vi "UI(Edit_Init).vi"(10 "Map":T1 {"TaskConfig"."SampleRateConfiguration"."SampleMode" items=["Finite Samples"=10178, "Continuous Samples"=10123, "Hardware Timed Single Point"=12522]}, 11 "Listbox":refnum<vi>) -> ()   [LabVIEW 2025, in "DAQ_Module.lvlib" / "DAQ_Module.lvclass"]
uses:
  DAQ_Module.lvclass
  DAQ_Config.ctl
  DAQ_Task_Config.ctl
  DAQ_HW_Type.ctl
  DAQ_Task_Type.ctl
  DAQ_SampleRateConfig.ctl
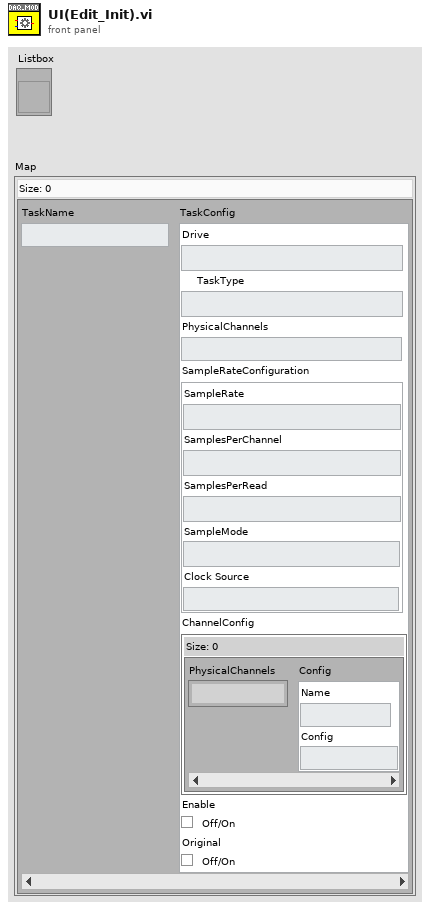
[diagram p1: front panel]
types:
  T1 = typedef "DAQ_Module.lvlib/DAQ_Module.lvclass/DAQ_Config.ctl" = map{string, T2}
  T2 = typedef "DAQ_Module.lvlib/DAQ_Module.lvclass/DAQ_Task_Config.ctl" = cluster{"Drive":T3, "TaskType":T4, "PhysicalChannels":string, "SampleRateConfiguration":T5, "ChannelConfig":map{string, cluster{"Name":string, "Config":string}}, "Enable":bool, "Original":bool}
  T3 = typedef "DAQ_Module.lvlib/DAQ_Module.lvclass/DAQ_HW_Type.ctl" = enum16{"NI_DAQmx", "Simulated_DAQ"}
  T4 = typedef "DAQ_Module.lvlib/DAQ_Module.lvclass/DAQ_Task_Type.ctl" = enum16{"AI", "Linear", "Angular", "AO"}
  T5 = typedef "DAQ_Module.lvlib/DAQ_Module.lvclass/DAQ_SampleRateConfig.ctl" = cluster{"SampleRate":dbl, "SamplesPerChannel":u32, "SamplesPerRead":i32, "SampleMode":i32, "Clock Source":string}
  T6 = cluster{"Left Cell String":string, "Child Text":string[], "Child Tag":string, "Item Indent":i32, "Child Only?":bool, "Glyph Index":i32}
  T7 = map{string, cluster{"Name":string, "Config":string}}
  T8 = cluster{"Left Cell String":string, "Child Text":string[], "Child Tag":string, "Item Indent":i32, "Child Only?":bool, "Glyph Index":i32}[]
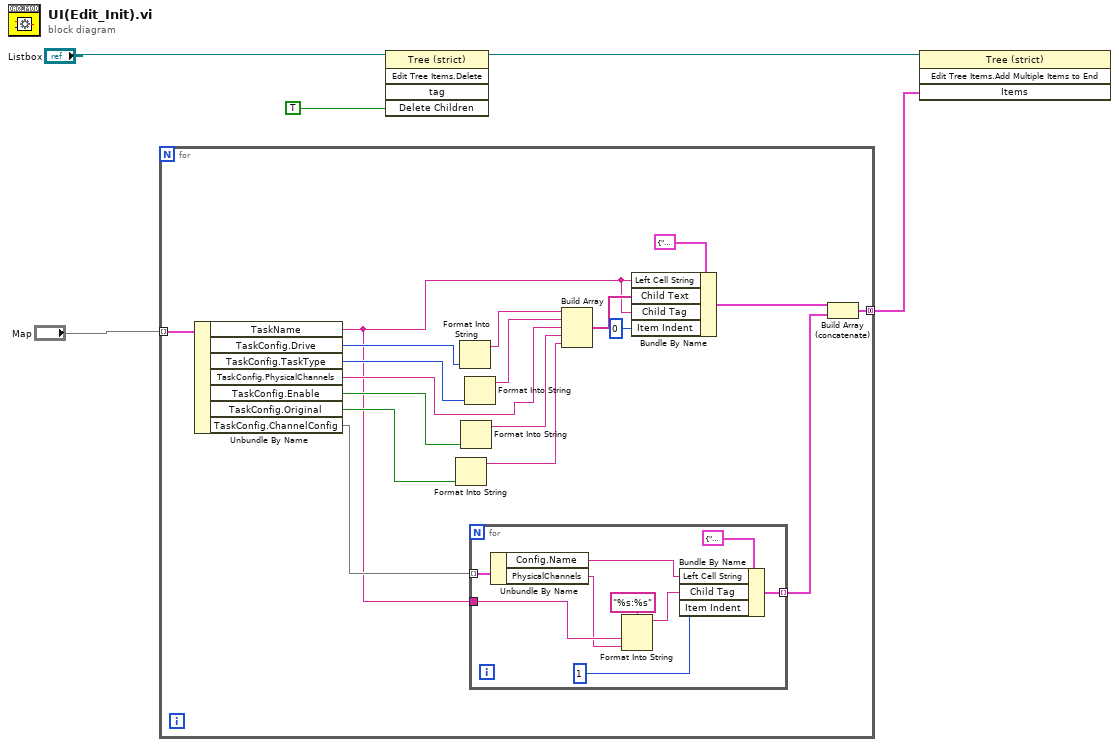
[diagram p0: block diagram]
diagram:
  n1 = for {
    tunnel: "Map" -> [w23] mode=indexing
    tunnel: [w6] -> w2 mode=concatenating
    n2 = Unbundle By Name(w23) -> ("TaskName"=w9:string, "TaskConfig.Drive"=w22:T3, "TaskConfig.TaskType"=w21:T4, "TaskConfig.PhysicalChannels"=w17:string, "TaskConfig.Enable"=w20:bool, "TaskConfig.Original"=w15:bool, "TaskConfig.ChannelConfig"=w11:T7)
    n3 = Format Into String(w15) -> (resulting string=w14:string)  [unwired: 3 in, 1 out]
    n4 = Format Into String(w22) -> (resulting string=w19:string)  [unwired: 3 in, 1 out]
    n5 = Format Into String(w20) -> (resulting string=w16:string)  [unwired: 3 in, 1 out]
    n6 = Format Into String(w21) -> (resulting string=w18:string)  [unwired: 3 in, 1 out]
    n7 = for {
      tunnel: w11 -> [w32] mode=indexing
      tunnel: w9 -> [w28]
      tunnel: [w25] -> w7 mode=indexing
      n8 = Unbundle By Name(w32) -> ("Config.Name"=w24:string, "PhysicalChannels"=w27:string)
      n9 = Format Into String(format string="%s:%s", w28, w27) -> (resulting string=w26:string)  [unwired: 2 in, 1 out]
      n10 = Bundle By Name(cluster=T6 {"Left Cell String"="", "Child Text"=[], "Child Tag"="", "Item Indent"=0, "Child Only?"=FALSE, "Glyph Index"=0} ("Item"), "Left Cell String"=w24, "Child Tag"=w26, "Item Indent"=1) -> (w25:T6)
    }
    n11 = Build Array(w19, w18, w17, w16, w14) -> (w12:string[])
    n12 = Bundle By Name(cluster=T6 {"Left Cell String"="", "Child Text"=[], "Child Tag"="", "Item Indent"=0, "Child Only?"=FALSE, "Glyph Index"=0} ("Item"), "Left Cell String"=w9, "Child Text"=w12, "Child Tag"=w9, "Item Indent"=0) -> (w8:T6)
    n13 = Build Array (concatenate)(w8, w7) -> (w6:T8)
  }
  n14 = invoke class="Tree (strict)" method="Edit Tree Items.Delete"(reference="Listbox", "Delete Children"=TRUE ("Delete Children?")) -> (reference out=w3:refnum<vi>)  [unwired: 3 in, 4 out]
  n15 = invoke class="Tree (strict)" method="Edit Tree Items.Add Multiple Items to End"(reference=w3, "Items"=w2) -> ()  [unwired: 2 in, 4 out]
